vi "EditorMain.vi"() -> ()   [LabVIEW 2018]
uses:
  ctl/dataGraphState.ctl
  ctl/editScriptState.ctl
  ctl/dataListboxState.ctl
  <vilib>/Utility/miscctls.llb/LVRowAndColumnTypeDef.ctl
  Class/EditorThumbnail.lvclass
panel:
  in  "add":bool
  in  "limit":T1={"plotIdx"=-1, "Minimum"=100.0, "Maximum"=900.0}
  in  "Script Btn":bool
  in  "Save As Button":bool
  in  "Open Button":bool
  out "XY Graph":cluster{"X":dbl[], "Y":sgl[]}[](graph)
  in  "Next Button":bool
  in  "Previous Button":bool
  in  "Shadow":bool
  in  "Array":T2(array[cluster])
  in  "mouseState":enum16{"idle", "down", "move", "up"}(ring)
  out "stop":bool
  out "updDataTrig":bool
  in  "InfoListbox":i32(listbox)=-1
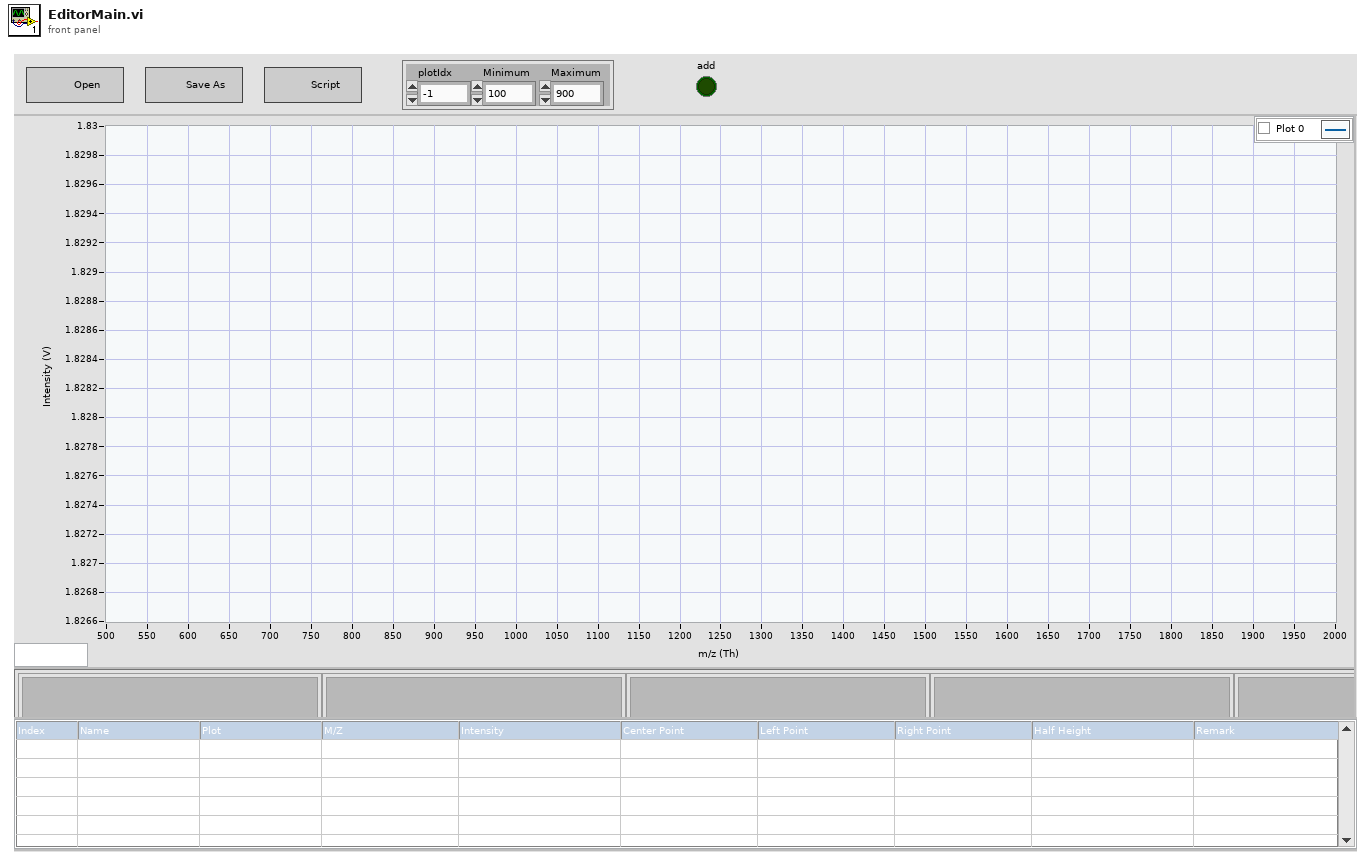
[diagram p1: front panel]
types:
  T1 = cluster{"plotIdx":i32, "Minimum":dbl, "Maximum":dbl}
  T2 = cluster{"index":u32, "data":cluster{"xdata":dbl[], "ydata":sgl[]}[], "peak":dbl[], "picture":picture}[]
  T3 = cluster{"graphRefnum":refnum<vi>, "shadowRefnum":refnum<vi>, "mouseState":refnum<vi>, "Previous Button":refnum<vi>, "Next Button":refnum<vi>, "thumbnailArrayRefnum":refnum<vi>, "topSpl":refnum<vi>, "bottomSpl":refnum<vi>}
  T4 = enum8{"Enabled", "Disabled", "Disabled and Grayed Out"}
  T5 = typedef "dataListboxState.ctl" = enum16{"init", "setData", "upd", "getExport"}
  T6 = typedef "editScriptState.ctl" = enum16{"init", "loadScript", "newScript", "runScript", "close"}
  T7 = typedef "dataGraphState.ctl" = enum16{"init", "set"}
  T8 = cluster{"startTime":dbl, "scanSig":cluster{"priDt":dbl, "priXData":dbl[], "priYData":sgl[], "beta":dbl[]}[], "listboxData":string[][]}
  T9 = cluster{"startTime":dbl, "scanData":cluster{"dt":dbl, "xdata":dbl[], "ydata":sgl[], "beta":dbl[]}[], "xyXLabel":string, "xyYLabel":string, "peakData":cluster{"xLeftIdx":u32[], "xCenterIdx":u32[], "xRightIdx":u32[], "baseline":sgl[], "halfHeight":dbl[]}[]}
  T10 = cluster{"dt":dbl, "xdata":dbl[], "ydata":sgl[], "beta":dbl[]}[]
  T11 = typedef "LVRowAndColumnTypeDef.ctl" = cluster{"Row":i32, "Column":i32}
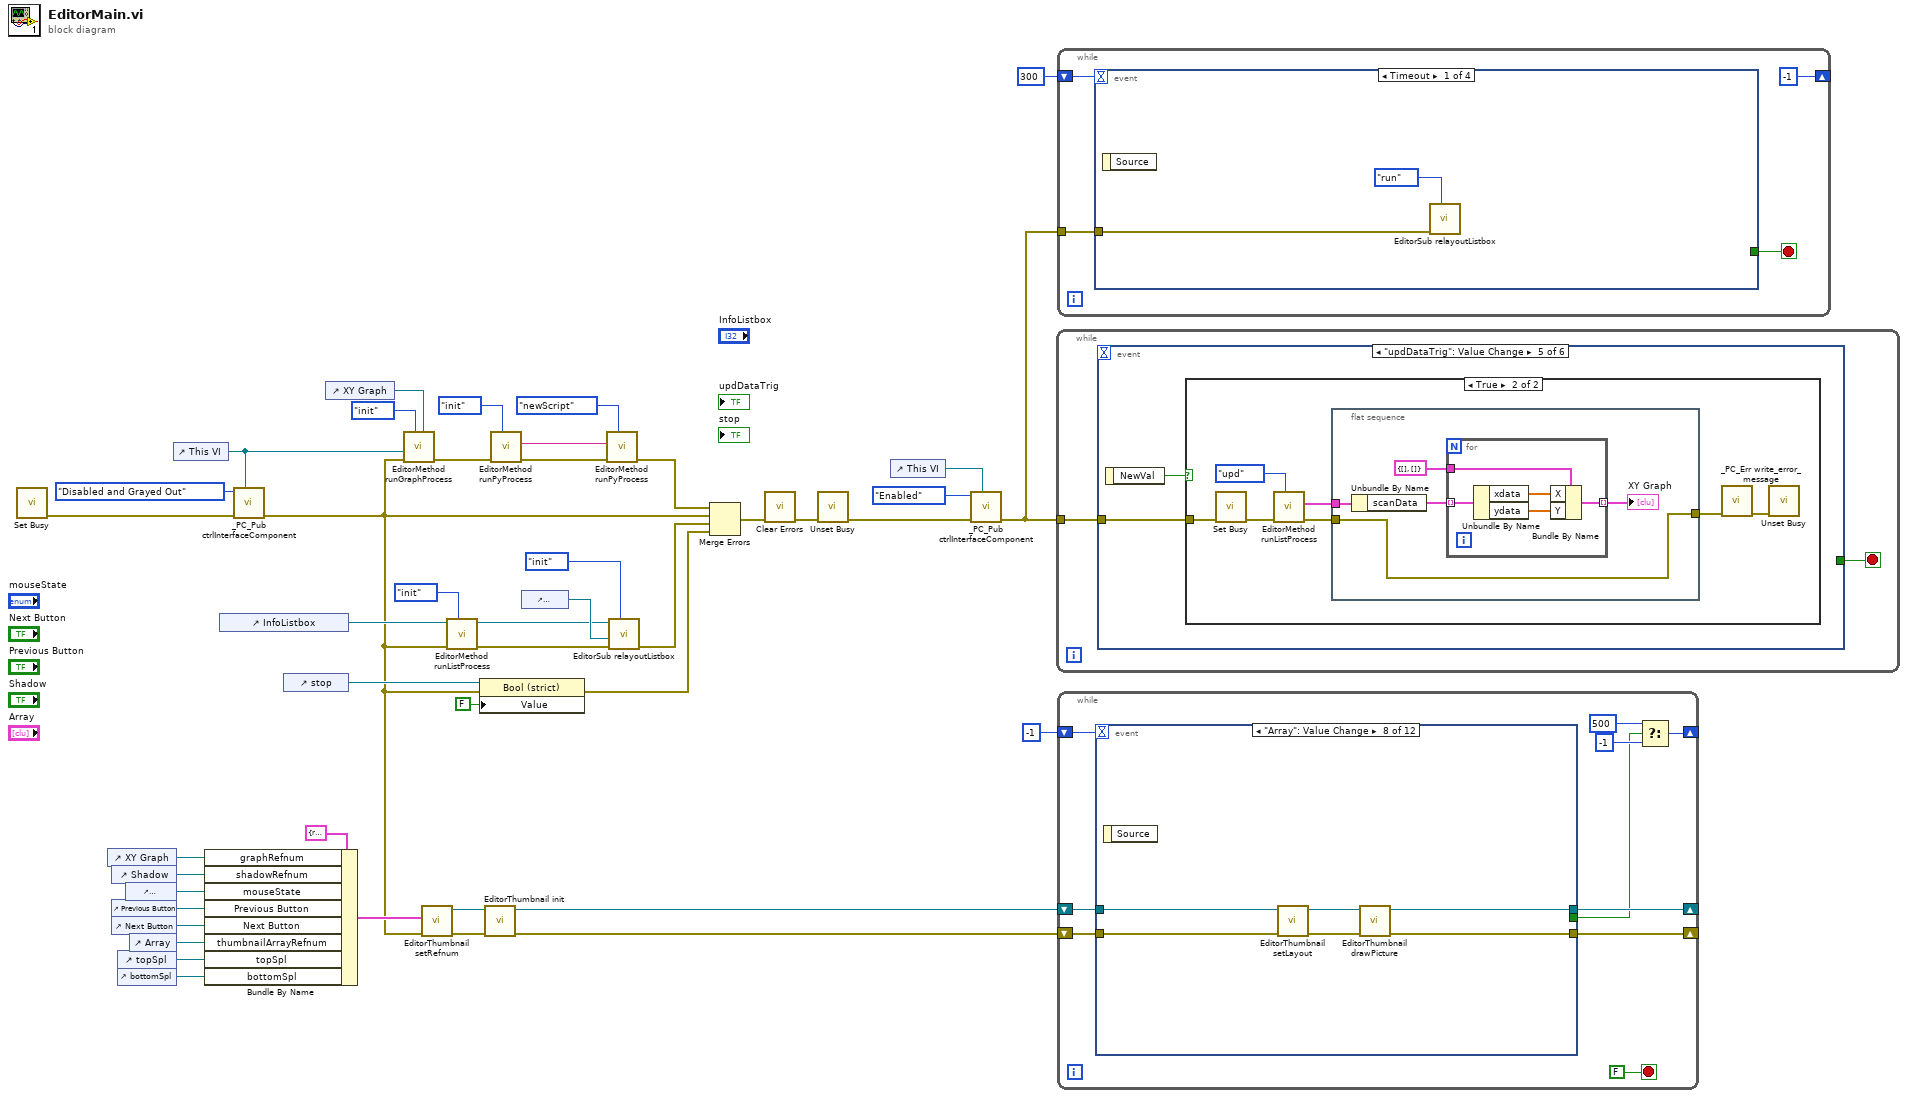
[diagram p0: block diagram]
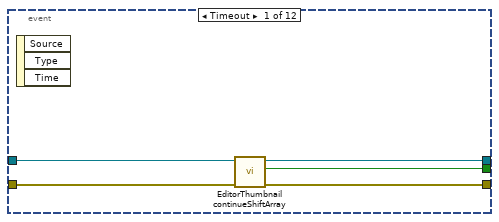
[diagram p2: hidden frame]
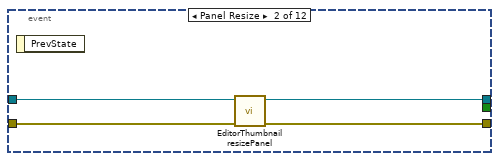
[diagram p3: hidden frame]
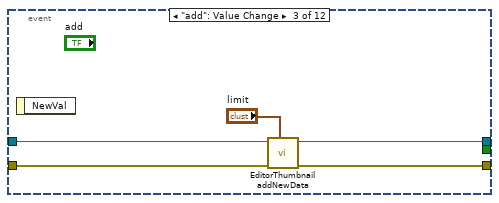
[diagram p4: hidden frame]
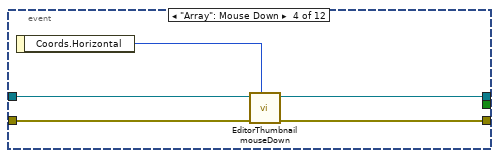
[diagram p5: hidden frame]
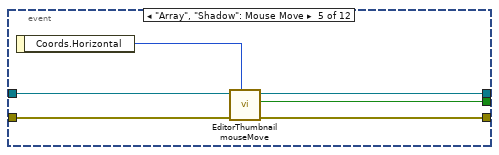
[diagram p6: hidden frame]
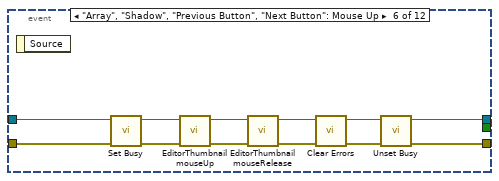
[diagram p7: hidden frame]
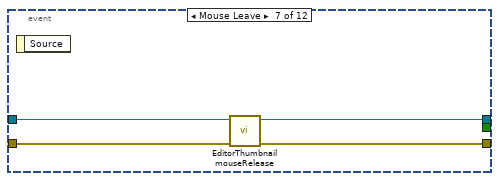
[diagram p8: hidden frame]
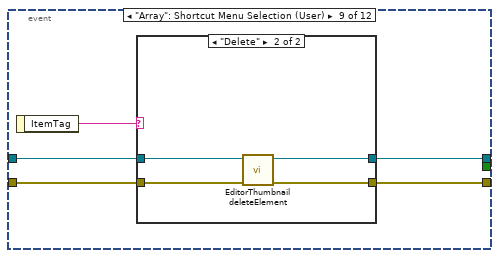
[diagram p9: hidden frame]
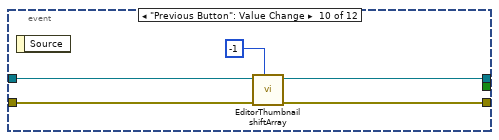
[diagram p11: hidden frame]
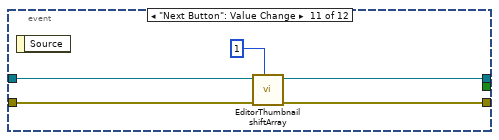
[diagram p12: hidden frame]
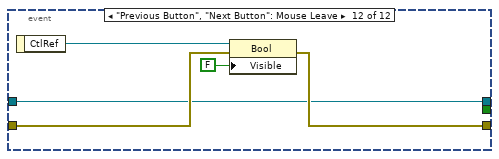
[diagram p13: hidden frame]
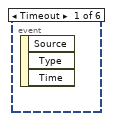
[diagram p14: hidden frame]
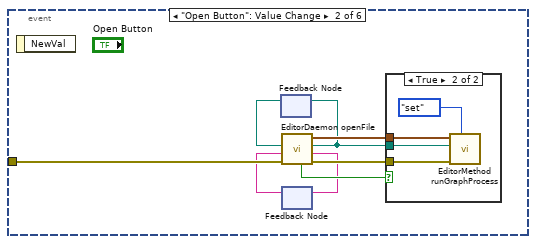
[diagram p15: hidden frame]
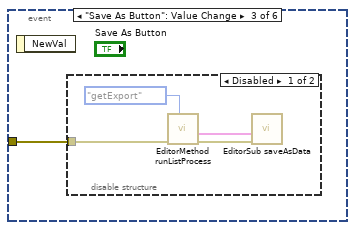
[diagram p17: hidden frame]
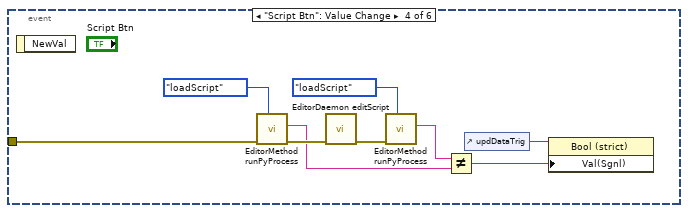
[diagram p19: hidden frame]
diagram:
  n1 = call <vilib>:"Set Busy.vi"() -> ("error out"=w22:errorcluster)  [unwired: 10 in, 1 out]
  n2 = control-ref of="XY Graph"() -> (w11:refnum<vi>)
  n3 = control-ref of="Shadow"() -> (w10:refnum<vi>)
  n4 = control-ref of="Previous Button"() -> (w8:refnum<vi>)
  n5 = control-ref of="Next Button"() -> (w7:refnum<vi>)
  n6 = control-ref of="topSpl"() -> (w5:refnum<vi>)
  n7 = control-ref of="bottomSpl"() -> (w4:refnum<vi>)
  n8 = control-ref of="mouseState"() -> (w9:refnum<vi>)
  n9 = control-ref of="Array"() -> (w6:refnum<vi>)
  n10 = control-ref of="This VI"() -> (w21:refnum<vi>)
  n11 = Bundle By Name(cluster=T3 {"graphRefnum"=refnum, "shadowRefnum"=refnum, "mouseState"=refnum, "Previous Button"=refnum, "Next Button"=refnum, "thumbnailArrayRefnum"=refnum, "topSpl"=refnum, "bottomSpl"=refnum} ("clusterRefnum"), "graphRefnum"=w11, "shadowRefnum"=w10, "mouseState"=w9, "Previous Button"=w8, "Next Button"=w7, "thumbnailArrayRefnum"=w6, "topSpl"=w5, "bottomSpl"=w4) -> (w3:T3)
  n12 = control-ref of="InfoListbox"() -> (w29:refnum<vi>)
  n13 = call "_PC_Pub ctrlInterfaceComponent.vi"("This VI"=w21, "error in (no error)"=w22, "Disabled"=T4."Disabled and Grayed Out") -> ("error out"=w1:errorcluster)  [unwired: 8 in]
  n14 = control-ref of="stop"() -> (w26:refnum<vi>)
  n15 = control-ref of="XY Graph"() -> (w42:refnum<vi>)
  n16 = call "EditorMethod runGraphProcess.vi"("xyGraphRefnum"=w42, "state"=dataGraphState."init", "error in (no error)"=w1, "This VI"=w21) -> ("error out"=w41:errorcluster)  [unwired: 7 in]
  n17 = call "EditorThumbnail setRefnum.vi"("error in (no error)"=w1, "clusterRefnum"=w3) -> ("error out"=w16:errorcluster, "EditorThumbnail out"=w17:refnum<class "EditorThumbnail.lvclass">)  [unwired: 8 in]
  n18 = call "EditorMethod runListProcess.vi"("state"=dataListboxState."init", "error in (no error)"=w1, "listboxRefnum"=w29) -> ("error out"=w30:errorcluster, "listboxRefnum out"=w31:refnum<vi>)  [unwired: 5 in, 2 out]
  n19 = property class="Bool (strict)"(reference=w26, error in=w1, "Value"=FALSE) -> (error out=w24:errorcluster)  [unwired: 1 out]
  n20 = call "EditorThumbnail init.vi"("error in (no error)"=w16, "EditThumbnail in"=w17) -> ("error out"=w14:errorcluster, "EditThumbnail out"=w13:refnum<class "EditorThumbnail.lvclass">)  [unwired: 8 in]
  n21 = call "EditorMethod runPyProcess.vi"("func"=editScriptState."init", "error in (no error)"=w41) -> ("error out"=w40:errorcluster, "pyCode"=w39:string)  [unwired: 6 in, 2 out]
  n22 = control-ref of="listboxPaneRefnum"() -> (w43:refnum<vi>)
  n23 = call "EditorMethod runPyProcess.vi"("func"=editScriptState."newScript", "error in (no error)"=w40, "newScriptCode"=w39) -> ("error out"=w38:errorcluster)  [unwired: 5 in, 3 out]
  n24 = call "EditorSub relayoutListbox.vi"("function"=enum16{"init", "run"}."init", "error in (no error)"=w30, "listboxPaneRefnum"=w43, "listboxRefnum"=w31) -> ("error out"=w37:errorcluster)  [unwired: 7 in]
  n25 = Merge Errors(w38, w1, w37, w24) -> (w36:errorcluster)
  n26 = call <vilib>:"Clear Errors.vi"("error in (no error)"=w36) -> ("error out"=w35:errorcluster)  [unwired: 5 in, 1 out]
  n27 = call <vilib>:"Unset Busy.vi"("error in (no error)"=w35) -> ("error out"=w18:errorcluster)  [unwired: 10 in]
  n28 = control-ref of="This VI"() -> (w19:refnum<vi>)
  n29 = call "_PC_Pub ctrlInterfaceComponent.vi"("This VI"=w19, "error in (no error)"=w18, "Disabled"=T4."Enabled") -> ("error out"=w15:errorcluster)  [unwired: 8 in]
  n30 = while {
    tunnel: w15 -> [w46]
    stop <- w45 stop-if-true
    n31 = event shown="[4] \"updDataTrig\": Value Change" {
      selector: _ -> [_ _ _ _ _ _]
      dyn-events: _ -> [_ _ _ _ _ _]
      timeout: _ -> [_ _ _ _ _ _]
      tunnel: w46 -> [_ w54 w59 w71 w74 _]
      tunnel: [_ _ _ _ _ w92] -> w45
      event Timeout {
        n32 = event-data() -> ()  [unwired: 1 in, 3 out]
      }
      event "Open Button": Value Change {
        n33 = event-data() -> ()  [unwired: 1 in, 1 out]
        n34 = feedback #1() -> (w51:path)  [unwired: 1 in]
        n35 = feedback #2() -> (w48:string)  [unwired: 1 in]
        n36 = call "EditorDaemon openFile.vi"("error in (no error)"=w54, "dataName"=w48, "filePath"=w51) -> ("error out"=w52:errorcluster, "dataName out"=w49:string, "currFilePath"=w47:path, "signal out"=w53:waveform(sgl), "update"=w50:bool)  [unwired: 4 in]
        n37 = feedback-in #1(w47) -> ()
        n38 = feedback-in #2(w49) -> ()
        n39 = case shown="True" w50 {
          tunnel: w53 -> [_ w58]
          tunnel: w52 -> [_ w57]
          tunnel: w47 -> [_ w55]
          frame False {
          }
          frame True {
            n40 = call "EditorMethod runGraphProcess.vi"("state"=dataGraphState."set", "error in (no error)"=w57, "currFilePath"=w55, "signal in"=w58) -> ()  [unwired: 7 in, 1 out]
          }
        }
      }
      event "Save As Button": Value Change {
        n41 = event-data() -> ()  [unwired: 1 in, 1 out]
        n42 = disable-structure shown="Disabled" {
          disable-tunnel: w59 -> [w62 _]
          frame Disabled {
            n43 = call "EditorMethod runListProcess.vi"("state"=dataListboxState."getExport", "error in (no error)"=w62) -> ("error out"=w60:errorcluster, "exportData"=w61:T8)  [unwired: 6 in, 2 out]
            n44 = call "EditorSub saveAsData.vi"("error in (no error)"=w60, "exportData"=w61) -> ()  [unwired: 9 in, 1 out]
          }
          frame Enabled {
          }
        }
      }
      event "Script Btn": Value Change {
        n45 = event-data() -> ()  [unwired: 1 in, 1 out]
        n46 = call "EditorMethod runPyProcess.vi"("func"=editScriptState."loadScript", "error in (no error)"=w71) -> ("error out"=w70:errorcluster, "pyCode"=w66:string)  [unwired: 6 in, 2 out]
        n47 = call "EditorDaemon editScript.vi"("error in (no error)"=w70) -> ("error out"=w68:errorcluster)  [unwired: 10 in]
        n48 = call "EditorMethod runPyProcess.vi"("func"=editScriptState."loadScript", "error in (no error)"=w68) -> ("pyCode"=w67:string)  [unwired: 6 in, 3 out]
        n49 = Not Equal?(x=w67, y=w66) -> (x != y?=w64:bool)
        n50 = control-ref of="updDataTrig"() -> (w65:refnum<vi>)
        n51 = property class="Bool (strict)"(reference=w65, "Val(Sgnl)"=w64) -> ()  [unwired: 1 in, 2 out]
      }
      event "updDataTrig": Value Change {
        n52 = event-data() -> ("NewVal"=w73:bool)  [unwired: 1 in]
        n53 = case shown="True" w73 {
          tunnel: w74 -> [_ w78]
          frame False {
          }
          frame True {
            n54 = call <vilib>:"Set Busy.vi"("error in (no error)"=w78) -> ("error out"=w77:errorcluster)  [unwired: 9 in, 1 out]
            n55 = call "EditorMethod runListProcess.vi"("state"=dataListboxState."upd", "error in (no error)"=w77) -> ("error out"=w79:errorcluster, "newSigInfo"=w80:T9)  [unwired: 6 in, 2 out]
            n56 = flat-sequence {
              tunnel: w80 -> [w84]
              tunnel: w79 -> [w82]
              tunnel: [w82] -> w76
              frame #0 {
                n57 = Unbundle By Name(w84) -> ("scanData"=w86:T10)
                n58 = for {
                  tunnel: w86 -> [w91] mode=indexing
                  tunnel: cluster{"X":dbl[], "Y":sgl[]} {"X"=[], "Y"=[]} ("Spectrum in") -> [w90]
                  tunnel: [w87] -> w83 mode=indexing
                  n59 = Unbundle By Name(w91) -> ("xdata"=w89:dbl[], "ydata"=w88:sgl[])
                  n60 = Bundle By Name(cluster=w90, "X"=w89, "Y"=w88) -> (w87:cluster{"X":dbl[], "Y":sgl[]})
                }
                "XY Graph" <- w83
              }
            }
            n61 = call "_PC_Err write_error_message.vi"("error in"=w76) -> ("error out"=w75:errorcluster)  [unwired: 10 in]
            n62 = call <vilib>:"Unset Busy.vi"("error in (no error)"=w75) -> ()  [unwired: 10 in, 1 out]
          }
        }
      }
      event "stop": Value Change {
        n63 = event-data() -> ("NewVal"=w92:bool)  [unwired: 1 in]
      }
    }
  }
  n64 = while {
    tunnel: w15 -> [w96]
    shift-right: [-1] -> _
    shift-left: 300 -> [w95]
    stop <- w93 stop-if-true
    n65 = event shown="[0] Timeout" {
      selector: _ -> [_ _ _ _]
      dyn-events: _ -> [_ _ _ _]
      timeout: w95 -> [_ _ _ _]
      tunnel: w96 -> [w97 w100 w101 w113]
      tunnel: [_ _ _ TRUE] -> w93
      event Timeout {
        n66 = event-data() -> ()  [unwired: 1 in, 1 out]
        n67 = call "EditorSub relayoutListbox.vi"("function"=enum16{"init", "run"}."run", "error in (no error)"=w97) -> ()  [unwired: 9 in, 1 out]
      }
      event Panel Resize {
        n68 = event-data() -> ()  [unwired: 1 in, 1 out]
        n69 = call "EditorSub relayoutListbox.vi"("function"=enum16{"init", "run"}."run", "error in (no error)"=w100) -> ()  [unwired: 9 in, 1 out]
      }
      event "InfoListbox": Mouse Down {
        n70 = event-data() -> ("CtlRef"=w102:refnum<vi>, "Mods.Double Click"=w103:bool)  [unwired: 1 in]
        n71 = case shown="True" w103 {
          tunnel: w102 -> [_ w111]
          tunnel: w101 -> [_ w104]
          frame False {
          }
          frame True {
            n72 = property class="MCListbox (strict)"(reference=w111, error in=w104) -> (reference out=w110:refnum<vi>, error out=w109:errorcluster, "Value"=w107:i32)
            n73 = Bundle By Name(cluster=T11 {"Row"=0, "Column"=0} ("Edit Position"), "Row"=w107, "Column"=9) -> (w106:T11)
            n74 = property class="MCListbox (strict)"(reference=w110, error in=w109, "EditPos"=w106) -> ()  [unwired: 2 out]
          }
        }
      }
      event Panel Close {
        n75 = event-data() -> ()  [unwired: 1 in, 1 out]
        n76 = control-ref of="stop"() -> (w114:refnum<vi>)
        n77 = property class="Bool (strict)"(reference=w114, error in=w113, "Val(Sgnl)"=TRUE ("Value (Signaling)")) -> ()  [unwired: 2 out]
      }
    }
  }
  n78 = while {
    shift-right: [w123] -> _
    shift-left: w13 -> [w124]
    shift-right: [w122] -> _
    shift-left: w14 -> [w125]
    shift-right: [w118] -> _
    shift-left: -1 -> [w119]
    stop <- FALSE stop-if-true
    n79 = event shown="[7] \"Array\": Value Change" {
      selector: _ -> [_ _ _ _ _ _ _ _ _ _ _ _]
      dyn-events: _ -> [_ _ _ _ _ _ _ _ _ _ _ _]
      timeout: w119 -> [_ _ _ _ _ _ _ _ _ _ _ _]
      tunnel: w125 -> [w129 w133 w138 w142 w145 w152 w162 w166 w173 w183 w188 w193]
      tunnel: w124 -> [w130 w134 w139 w143 w149 w154 w163 w167 w174 w184 w189 w191]
      tunnel: [w126 w131 w137 w140 w148 w153 w160 w165 w172 w181 w186 w191] -> w123
      tunnel: [w128 w132 w136 w141 w146 w151 w161 w164 w171 w182 w187 w192] -> w122
      tunnel: [w127 _ _ _ w147 _ _ _ _ _ _ _] -> w117
      event Timeout {
        n80 = event-data() -> ()  [unwired: 1 in, 3 out]
        n81 = call "EditorThumbnail continueShiftArray.vi"("error in (no error)"=w129, "EditorThumbnail in"=w130) -> ("error out"=w128:errorcluster, "Timing"=w127:bool, "EditorThumbnail out"=w126:refnum<class "EditorThumbnail.lvclass">)  [unwired: 7 in]
      }
      event Panel Resize {
        n82 = event-data() -> ()  [unwired: 1 in, 1 out]
        n83 = call "EditorThumbnail resizePanel.vi"("error in (no error)"=w133, "EditorThumbnail in"=w134) -> ("error out"=w132:errorcluster, "EditorThumbnail out"=w131:refnum<class "EditorThumbnail.lvclass">)  [unwired: 8 in]
      }
      event "add": Value Change {
        n84 = event-data() -> ()  [unwired: 1 in, 1 out]
        n85 = call "EditorThumbnail addNewData.vi"("limit"="limit", "error in (no error)"=w138, "EditorThumbnail in"=w139) -> ("error out"=w136:errorcluster, "EditorThumbnail out"=w137:refnum<class "EditorThumbnail.lvclass">)  [unwired: 7 in]
      }
      event "Array": Mouse Down {
        n86 = event-data() -> ("Coords.Horizontal"=w144:i32)  [unwired: 1 in]
        n87 = call "EditorThumbnail mouseDown.vi"("coordsHorizontal"=w144, "error in (no error)"=w142, "EditorThumbnail in"=w143) -> ("error out"=w141:errorcluster, "EditorThumbnail out"=w140:refnum<class "EditorThumbnail.lvclass">)  [unwired: 6 in, 1 out]
      }
      event "Array", "Shadow": Mouse Move {
        n88 = event-data() -> ("Coords.Horizontal"=w150:i32)  [unwired: 1 in]
        n89 = call "EditorThumbnail mouseMove.vi"("coordsHorizontal"=w150, "error in (no error)"=w145, "EditorThumbnail in"=w149) -> ("error out"=w146:errorcluster, "Timing"=w147:bool, "EditorThumbnail out"=w148:refnum<class "EditorThumbnail.lvclass">)  [unwired: 6 in]
      }
      event "Array", "Shadow", "Previous Button", "Next Button": Mouse Up {
        n90 = event-data() -> ()  [unwired: 1 in, 1 out]
        n91 = call <vilib>:"Set Busy.vi"("error in (no error)"=w152) -> ("error out"=w159:errorcluster)  [unwired: 9 in, 1 out]
        n92 = call "EditorThumbnail mouseUp.vi"("error in (no error)"=w159, "EditorThumbnail in"=w154) -> ("error out"=w155:errorcluster, "EditorThumbnail out"=w156:refnum<class "EditorThumbnail.lvclass">)  [unwired: 8 in]
        n93 = call "EditorThumbnail mouseRelease.vi"("error in (no error)"=w155, "EditorThumbnail in"=w156) -> ("error out"=w158:errorcluster, "EditorThumbnail out"=w153:refnum<class "EditorThumbnail.lvclass">)  [unwired: 8 in]
        n94 = call <vilib>:"Clear Errors.vi"("error in (no error)"=w158) -> ("error out"=w157:errorcluster)  [unwired: 5 in, 1 out]
        n95 = call <vilib>:"Unset Busy.vi"("error in (no error)"=w157) -> ("error out"=w151:errorcluster)  [unwired: 10 in]
      }
      event Mouse Leave {
        n96 = event-data() -> ()  [unwired: 1 in, 1 out]
        n97 = call "EditorThumbnail mouseRelease.vi"("error in (no error)"=w162, "EditorThumbnail in"=w163) -> ("error out"=w161:errorcluster, "EditorThumbnail out"=w160:refnum<class "EditorThumbnail.lvclass">)  [unwired: 8 in]
      }
      event "Array": Value Change {
        n98 = event-data() -> ()  [unwired: 1 in, 1 out]
        n99 = call "EditorThumbnail setLayout.vi"("error in (no error)"=w166, "EditorThumbnail in"=w167) -> ("error out"=w168:errorcluster, "EditorThumbnail out"=w169:refnum<class "EditorThumbnail.lvclass">)  [unwired: 8 in]
        n100 = call "EditorThumbnail drawPicture.vi"("error in (no error)"=w168, "EditorThumbnail in"=w169) -> ("error out"=w164:errorcluster, "EditorThumbnail out"=w165:refnum<class "EditorThumbnail.lvclass">)  [unwired: 8 in]
      }
      event "Array": Shortcut Menu Selection (User) {
        n101 = event-data() -> ("ItemTag"=w170:string)  [unwired: 1 in]
        n102 = case shown="\"Delete\"" w170 {
          tunnel: w174 -> [w176 w180]
          tunnel: w173 -> [w175 w177]
          tunnel: [w175 w178] -> w171
          tunnel: [w176 w179] -> w172
          frame Default {
          }
          frame "Delete" {
            n103 = call "EditorThumbnail deleteElement.vi"("error in (no error)"=w177, "EditorThumbnail in"=w180) -> ("error out"=w178:errorcluster, "EditorThumbnail out"=w179:refnum<class "EditorThumbnail.lvclass">)  [unwired: 8 in]
          }
        }
      }
      event "Previous Button": Value Change {
        n104 = event-data() -> ()  [unwired: 1 in, 1 out]
        n105 = call "EditorThumbnail shiftArray.vi"("add"=-1, "error in (no error)"=w183, "EditorThumbnail in"=w184) -> ("error out"=w182:errorcluster, "EditorThumbnail out"=w181:refnum<class "EditorThumbnail.lvclass">)  [unwired: 7 in]
      }
      event "Next Button": Value Change {
        n106 = event-data() -> ()  [unwired: 1 in, 1 out]
        n107 = call "EditorThumbnail shiftArray.vi"("add"=1, "error in (no error)"=w188, "EditorThumbnail in"=w189) -> ("error out"=w187:errorcluster, "EditorThumbnail out"=w186:refnum<class "EditorThumbnail.lvclass">)  [unwired: 7 in]
      }
      event "Previous Button", "Next Button": Mouse Leave {
        n108 = event-data() -> ("CtlRef"=w194:refnum<vi>)  [unwired: 1 in]
        n109 = property class="Bool"(reference=w194, error in=w193, "Visible"=FALSE) -> (error out=w192:errorcluster)  [unwired: 1 out]
      }
    }
    n110 = Select(t=500, s=w117, f=-1) -> (s? t:f=w118:i32)
  }
